vi "Configure Thermistor [THM].vi"(8 "error in (no error)":errorcluster, 10 "resistance (0.0 ohms)":dbl format="%^.2e", 11 "CS++DMM in":refnum<class "CS++DMM.lvclass">) -> (0 "error out":errorcluster, 3 "CS++DMM out":refnum<class "CS++DMM.lvclass">)   [LabVIEW 2013, in "CS++DMM.lvlib" / "CS++DMM.lvclass"]
doc: "This VI configures the resistance for a thermistor temperature measurement device.\n\nThis VI affects the behavior of the instrument only when the IviDmm>Temperature Measurements>Transducer Type [TMP] property is set to IVIDMM_VAL_THERMISTOR.\n\nNote:\n\n(1) This VI is part of the IviDmmThermistor [THM] extension group."
uses:
  CS++DMM.lvclass
  CSPP_Core/Classes/CS++ProcessVariables/ProcessVariable/PV.lvclass
  PV-Enum.ctl
  CSPP_Core/Classes/CS++ProcessVariables/ProcessVariable/PV.lvclass/PV.ctl
  CS++DMM.lvclass/CS++DMM.ctl
  CSPP_Core/Classes/CS++ProcessVariables/PVConnection/PVConnection.lvclass
  CSPP_Core/Classes/CS++ProcessVariables/ProcessVariable/Write Data.vi
  CSPP_Core/Classes/CS++ProcessVariables/ProcessVariable/Write Timestamp.vi
  CSPP_Core/Classes/CS++ProcessVariables/ProcessVariable/Write Quality.vi
  CSPP_Core/Classes/CS++ProcessVariables/ProcessVariable/Write status.vi
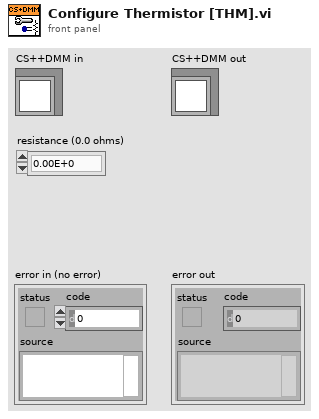
[diagram p1: front panel]
types:
  T1 = typedef "CS++DMM.lvlib/CS++DMM.lvclass/PV-Enum.ctl" = enum16{"AbsoluteResolution", "ACMaxFrequency", "ACMinFrequency", "ActualRange", "Alpha", "ApertureTime", "FixedReferenceJunction", "FrequencyVoltageRange", "PowerLineFrequency", "Range", "Reading", "Resistance", "SampleInterval", "TriggerDelay", "ApertureTimeUnit", "AutoZeroMode", "MeasCompleteDestination", "MeasurementFunction", "ReferenceJunctionType", "SampleCount", "SampleTrigger", "ThermocoupleType", "TranducerType", "TriggerCount", "TriggerSlope", "TriggerSource", "MPReading", "IsOverRange"}
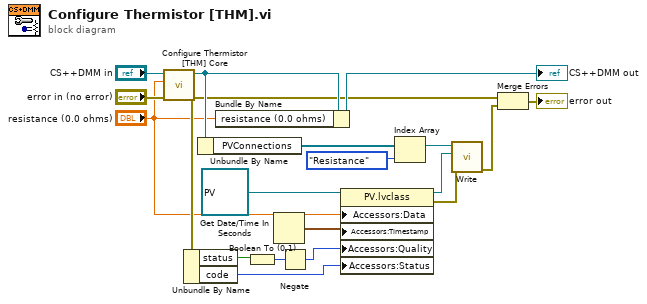
[diagram p0: block diagram]
diagram:
  n1 = call-dynamic "Configure Thermistor [THM] Core.vi"("error in (no error)"="error in (no error)", "resistance (0.0 ohms)"="resistance (0.0 ohms)", "CS++DMM in"="CS++DMM in") -> ("error out"=w6:errorcluster, "CS++DMM out"=w7:refnum<class "CS++DMM.lvclass">)  [unwired: 7 in]
  n2 = Unbundle By Name(w6) -> ("status"=w15:bool, "code"=w12:i32)
  n3 = Unbundle By Name(w7) -> ("PVConnections"=w10:refnum<class "PVConnection.lvclass">[])
  n4 = Bundle By Name(cluster=w7, "resistance (0.0 ohms)"="resistance (0.0 ohms)") -> (→"CS++DMM out":refnum<class "CS++DMM.lvclass">)
  n5 = Boolean To (0,1)(Boolean=w15) -> (0, 1=w14:i16)
  n6 = Get Date/Time In Seconds() -> (seconds since 1Jan1904=w11:timestamp)
  n7 = Negate(x=w14) -> (-x=w13:i16)
  n8 = property class="PV.lvclass"(reference=refnum<class "PV.lvclass"> refnum ("CS++ProcessVariables.lvlib:PV.lvclass"), "Accessors:Data"="resistance (0.0 ohms)", "Accessors:Timestamp"=w11, "Accessors:Quality"=w13, "Accessors:Status"=w12) -> (reference out=w9:refnum<class "PV.lvclass">, error out=w8:errorcluster)  [unwired: 1 in]
  n9 = Index Array(array=w10, index=PV-Enum."Resistance" ("PV-Enum")) -> (element=w2:refnum<class "PVConnection.lvclass">)
  n10 = call-dynamic "Write.vi"("error in (no error)"=w8, "PV"=w9, "PVConnection in"=w2) -> ("error out"=w3:errorcluster)  [unwired: 7 in, 1 out]
  n11 = Merge Errors(w6, w3) -> (→"error out":errorcluster)
